vi "StateNode_Create.vi"(0 "reference":refnum<class "ChoiceNode.lvclass">, 5 "error in (no error)":errorcluster, 6 "GoopReferenceIn":T1) -> (14 "reference out":refnum<class "ChoiceNode.lvclass">, 16 "# of objects":i32, 19 "error out":errorcluster)   [LabVIEW 2012, in "ChoiceNode.lvclass"]
doc: "Creates and initializes a new StateNode object.\n\nThis object should be destroyed using a StateNode destructor VI or a virtual base class destructor VI.\n\n[GOOP 2.1]"
uses:
  <resource>/Framework/Providers/Open_GDS/UML/ChoiceNode_class/ChoiceNode.lvclass
  <resource>/Framework/Providers/Open_GDS/UML/AbstractNode_class/ObjectReference.ctl
  <resource>/Framework/Providers/Open_GDS/UML/MultiLineString_class/SizeType.ctl
  <resource>/Framework/Providers/Open_GDS/UML/General/Rectangle/Rectangle Rectangle2D.ctl
  <resource>/Framework/Providers/Open_GDS/UML/MultiLineString_class/JustificationType.ctl
  <resource>/Framework/Providers/Open_GDS/UML/MultiLineString_class/MultiLineString.lvclass
  <resource>/Framework/Providers/Open_GDS/UML/RectangularNode_class/RectangularNode.lvclass
  <resource>/Framework/Providers/Open_GDS/UML/AbstractNode_class/AbstractNode.lvclass
panel:
  # "The input reference should only\nbe wired when this method is called\nby a sub class constructor."
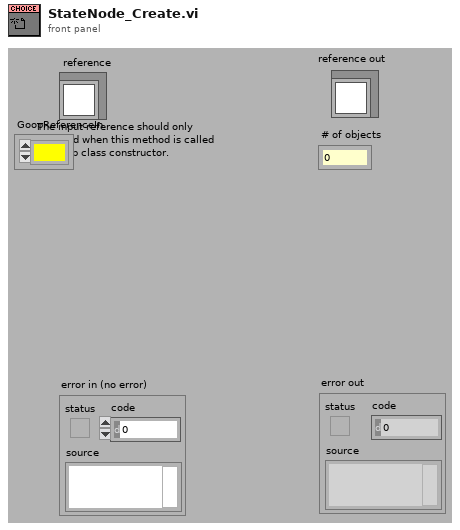
[diagram p1: front panel]
types:
  T1 = typedef "AbstractNode.lvclass/ObjectReference.ctl" = refnum<k1>
  T2 = typedef "MultiLineString.lvclass/JustificationType.ctl" = enum16{"LEFT", "CENTER", "RIGHT"}
  T3 = typedef "Rectangle Rectangle2D.ctl" = cluster{"x":dbl, "y":dbl, "width":dbl, "height":dbl}
  T4 = typedef "MultiLineString.lvclass/SizeType.ctl" = enum16{"LARGE", "NORMAL", "SMALL"}
  T5 = typedef "ChoiceNode.lvclass/ObjectAttributes.ctl" = cluster{"Base class":T6, "Text":refnum<class "MultiLineString.lvclass">, "DEFAULT_WIDTH":i32, "DEFAULT_HEIGHT":i32}
  T6 = typedef "RectangularNode.lvclass/ObjectAttributes.ctl" = cluster{"Base class":T7, "bounds":T3}
  T7 = typedef "AbstractNode.lvclass/ObjectAttributes.ctl" = cluster{"parent":refnum<class "AbstractNode.lvclass">, "children":refnum<class "AbstractNode.lvclass">[], "Hidden":bool}
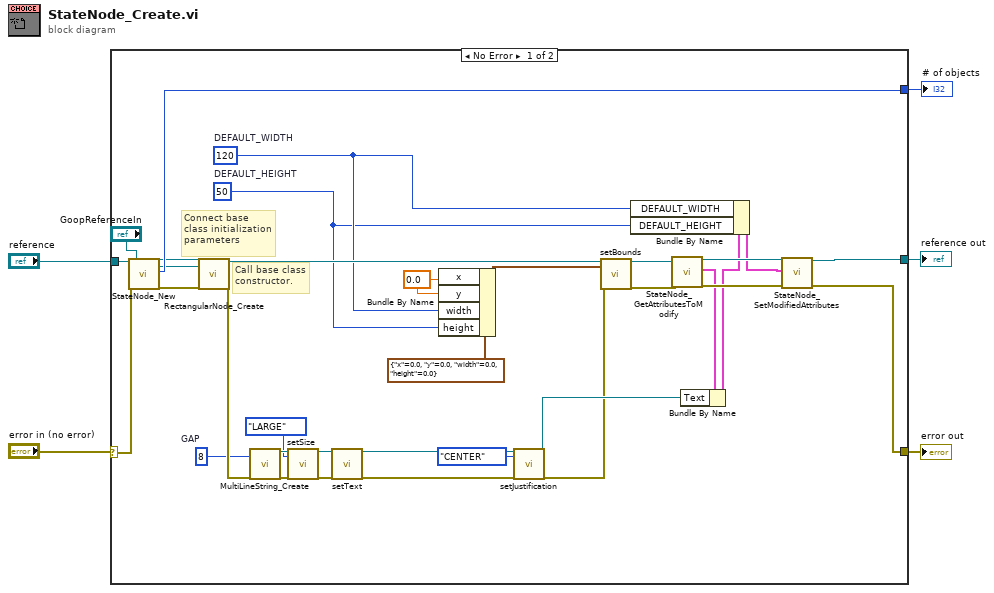
[diagram p0: block diagram]
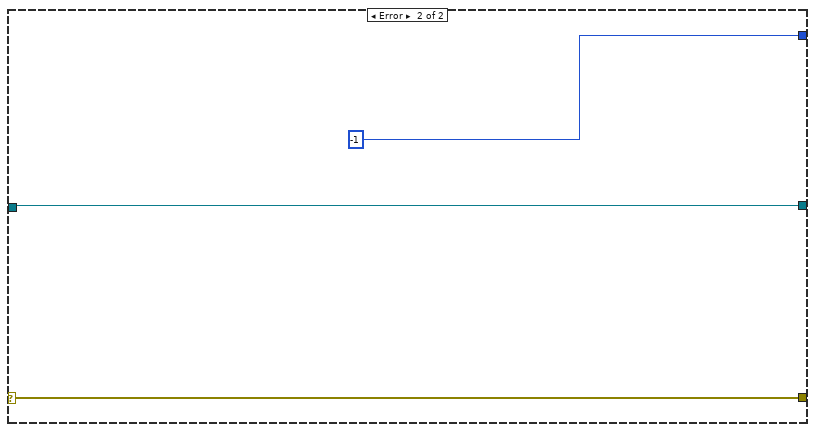
[diagram p2: hidden frame]
diagram:
  n1 = case shown="No Error" "error in (no error)" {
    selector: "error in (no error)" -> [w39 w41]
    tunnel: [w34 w40] -> w5
    tunnel: [w33 w41] -> w4
    tunnel: [w38 -1 ("Nr of open handles")] -> w3
    tunnel: "reference" -> [w37 w40]
    frame No Error {
      w24 = 0.0 ("x")
      w10 = 8  # GAP
      w22 = 50  # DEFAULT_HEIGHT
      w23 = 120  # DEFAULT_WIDTH
      # "Connect base\nclass initialization\nparameters"
      # "Call base class\nconstructor."
      n2 = call <resource>:"StateNode_New.vi"("reference in"=w37, "error in (no error)"=w39, "GoopReferenceIn"="GoopReferenceIn") -> ("GoopReferenceOut"=w8:T1, "reference out"=w21:refnum<class "ChoiceNode.lvclass">, "# of objects"=w38:i32, "error out"=w32:errorcluster)  [unwired: 2 in, 11 out]
      n3 = call <resource>:"RectangularNode_Create.vi"("reference"=w21, "error in (no error)"=w32, "GoopReferenceIn"=w8) -> ("reference out"=w27:refnum<class "ChoiceNode.lvclass">, "error out"=w11:errorcluster)  [unwired: 15 out]
      n4 = call <resource>:"MultiLineString_Create.vi"("GAP"=w10, "error in (no error)"=w11) -> ("reference out"=w31:refnum<class "MultiLineString.lvclass">, "error out"=w30:errorcluster)  [unwired: 2 in, 14 out]
      n5 = call <resource>:"setSize.vi"("reference"=w31, "size"=SizeType."LARGE", "error in (no error)"=w30) -> ("reference out"=w18:refnum<class "MultiLineString.lvclass">, "error out"=w17:errorcluster)  [unwired: 15 out]
      n6 = call-dynamic "setText.vi"("reference"=w18, "error in (no error)"=w17) -> ("reference out"=w13:refnum<class "MultiLineString.lvclass">, "error out"=w14:errorcluster)  [unwired: 16 in]
      n7 = Bundle By Name(cluster=T3 {"x"=0.0, "y"=0.0, "width"=0.0, "height"=0.0} ("bounds"), "x"=w24, "y"=w24, "width"=w23, "height"=w22) -> (w26:T3)
      n8 = call <resource>:"setJustification.vi"("reference"=w13, "justification"=JustificationType."CENTER", "error in (no error)"=w14) -> ("reference out"=w12:refnum<class "MultiLineString.lvclass">, "error out"=w6:errorcluster)  [unwired: 15 out]
      n9 = call-dynamic "setBounds.vi"("reference"=w27, "bounds"=w26, "error in (no error)"=w6) -> ("reference out"=w7:refnum<class "ChoiceNode.lvclass">, "error out"=w19:errorcluster)  [unwired: 15 in]
      n10 = call <resource>:"StateNode_GetAttributesToModify.vi"("reference in"=w7, "error in (no error)"=w19) -> ("reference out"=w35:refnum<class "ChoiceNode.lvclass">, "Attributes"=w20:T5, "error out"=w36:errorcluster)  [unwired: 1 in, 14 out]
      n11 = Bundle By Name(cluster=w20, "Text"=w12) -> (w16:T5)
      n12 = Bundle By Name(cluster=w16, "DEFAULT_WIDTH"=w23, "DEFAULT_HEIGHT"=w22) -> (w15:T5)
      n13 = call <resource>:"StateNode_SetModifiedAttributes.vi"("reference in"=w35, "Attributes"=w15, "error in (no error)"=w36) -> ("reference out"=w34:refnum<class "ChoiceNode.lvclass">, "error out"=w33:errorcluster)  [unwired: 3 in, 12 out]
    }
    frame Error {
    }
  }
  "error out" <- w4
  "reference out" <- w5
  "# of objects" <- w3
